vi "auto caps.vi"() -> ()   [LabVIEW 2014]
panel:
  in  "String":string
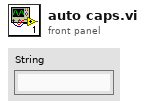
[diagram p1: front panel]
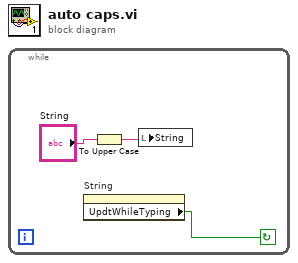
[diagram p0: block diagram]
diagram:
  n1 = while {
    stop <- w1 continue-if-true
    n2 = property on="String" class="Str"() -> ("UpdtWhileTyping"=w1:bool)  [unwired: 2 in, 2 out]
    n3 = To Upper Case(1:"String") -> (0:w2:string)
    n4 = local write "String"(w2) -> ()
  }
